vi "E03_for.vi"() -> ()   [LabVIEW 2026]
panel:
  out "Waveform Chart":dbl(graph)
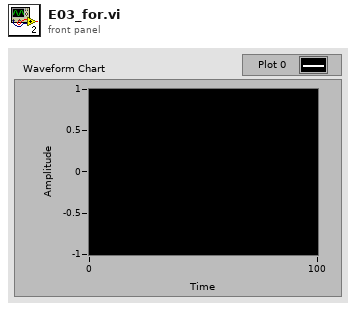
[diagram p1: front panel]
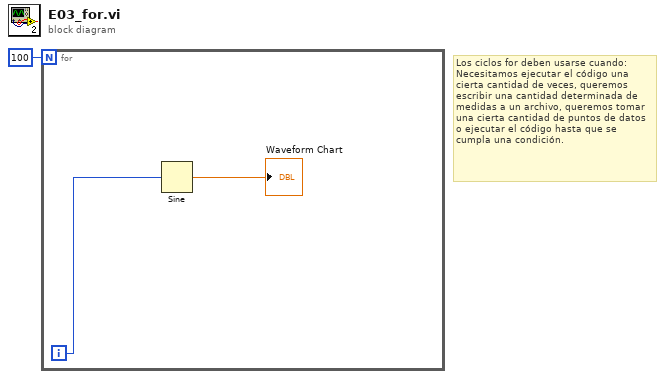
[diagram p0: block diagram]
diagram:
  # "Los ciclos for deben usarse cuando: Necesitamos ejecutar el código una cierta cantidad de veces, queremos escribir una cantidad determinada de medidas a un archivo, queremos tomar una cierta cantidad de puntos de datos o ejecutar el código hasta que se cumpla una condición."
  n1 = for {
    N: 100 -> [_]
    i -> [w3]
    n2 = Sine(x=w3) -> (sin(x)=→"Waveform Chart":dbl)
  }
